vi "Set Application Settings.vi"(8 "error in (no error)":errorcluster, 10 "Application Information":T1, 11 "BLF File In":refnum<class "Read Write BLF.lvclass">) -> (0 "error out":errorcluster, 3 "BLF File Out":refnum<class "Read Write BLF.lvclass">)   [LabVIEW 2015, in "Read Write BLF.lvclass"]
doc: "This VI will set the <B>Application Information</B> which states what application and what version, is writing the BLF file.\n\n-------------\nBrian Hoover (Hooovahh)"
uses:
  Read Write BLF.lvclass
  Controls/Cluster - Application Information.ctl
  Controls/Enum - Application ID.ctl
  Read Write BLF.lvclass/Read Write BLF.ctl
  <vilib>/Utility/error.llb/Error Cluster From Error Code.vi
  <vilib>/Utility/file.llb/Application Directory.vi
  <vilib>/ErrorRing/Error Ring.xnode
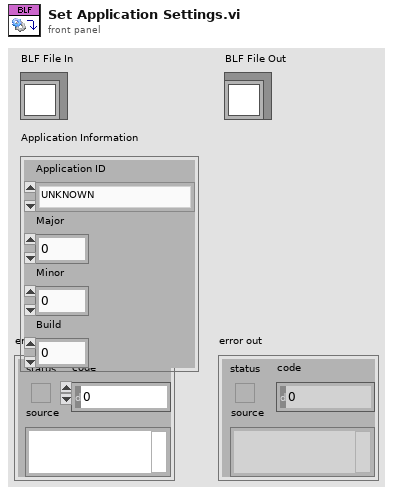
[diagram p1: front panel]
types:
  T1 = typedef "Read Write BLF.lvclass/Cluster - Application Information.ctl" = cluster{"Application ID":T2, "Major":u8, "Minor":u8, "Build":u8}
  T2 = typedef "Read Write BLF.lvclass/Enum - Application ID.ctl" = enum8{"UNKNOWN", "CANALYZER", "CANOE", "CANSTRESS", "CANLOG", "CANAPE", "CANCASEXLLOG"}
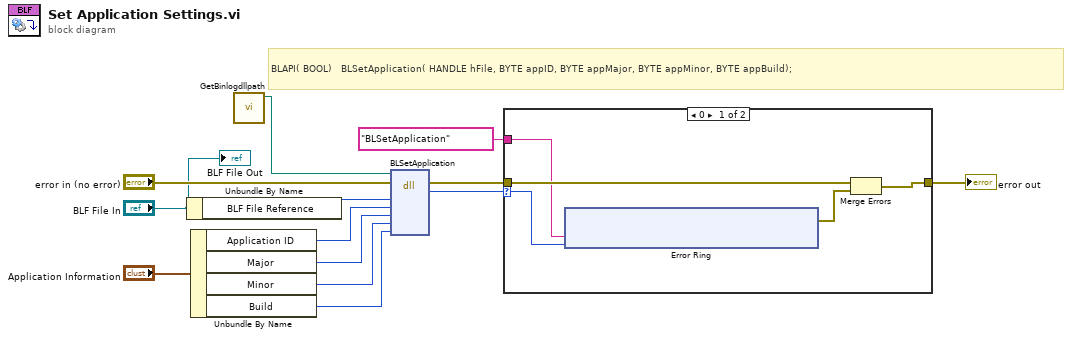
[diagram p0: block diagram]
diagram:
  # "BLAPI( BOOL)   BLSetApplication( HANDLE hFile, BYTE appID, BYTE appMajor, BYTE appMinor, BYTE appBuild);"
  n1 = Unbundle By Name("BLF File In") -> ("BLF File Reference"=w7:u32)
  n2 = Unbundle By Name("Application Information") -> ("Application ID"=w5:T2, "Major"=w4:u8, "Minor"=w3:u8, "Build"=w2:u8)
  n3 = call "GetBinlogdllpath.vi"() -> ("dup path"=w1:path)  [unwired: 11 in]
  n4 = dll-call lib="PTH2Vabs E自开发软件X-CAN项目 X-CAN离线分析平台 V2.2.8.0BLFbinlog.*" fn="BLSetApplication"(path in=w1, error in="error in (no error)", "hFile"=w7, "appID"=w5, "appMajor"=w4, "appMinor"=w3, "appBuild"=w2) -> (error out=w9:errorcluster, "return type"=w11:i32)  [unwired: 6 in, 1 out]
  n5 = case shown="0" w11 {
    selector: w11 -> [w16 _]
    tunnel: w9 -> [w18 w27]
    tunnel: [w17 w27] -> w10
    tunnel: "BLSetApplication" -> [w15 _]
    frame 0 {
      n6 = xnode "Error Ring"("参数 0"=w15, "参数 1"=w16) -> ("错误输出"=w14:errorcluster)
      n7 = Merge Errors(w18, w14) -> (w17:errorcluster)
    }
    frame Default {
    }
  }
  "error out" <- w10
  "BLF File Out" <- "BLF File In"
